vi "创建企业.vi"(9 "企业信息":T2, 11 "数据库操作.i":refnum<class "数据库操作.lvclass">) -> (1 "删除企业成功？":bool, 2 "创建结果":string caption="结果", 3 "数据库操作.o":refnum<class "数据库操作.lvclass">)   [LabVIEW 2013, in "数据库操作.lvclass"]
uses:
  <vilib>/addons/database/Connection.llb/Conn Execute.vi
  <vilib>/Utility/config.llb/Write Key (String).vi
  <vilib>/Utility/config.llb/NI_LVConfig.lvlib
  <vilib>/addons/database/NI_Database_API.lvlib
panel:
  out "剂量统计":enum16{"用户名", "年", "月", "周", "日", "剂量"}(ring)
  out "用户列表":T1(ring)
  out "企业信息.ini":enum16{"登录名", "密码", "企业名称", "邮箱", "电话"}(ring)
  # "字段参考"
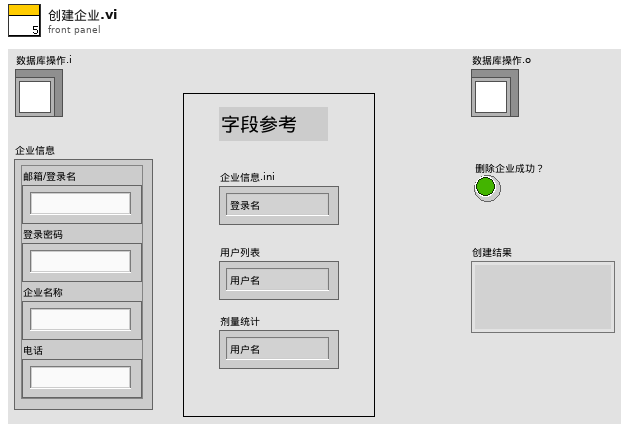
[diagram p1: front panel]
types:
  T1 = enum16{"用户名", "设备MAC", "设备状态", "密码", "职类", "姓名", "电话", "邮箱", "备注", "最后活动"}
  T2 = cluster{"邮箱/登录名":string, "登录密码":string, "企业名称":string, "电话":string}
  T3 = typedef "NI_Database_API.lvlib/Conn ObjectReference.ctl" = refnum<k1>
  T4 = typedef "NI_LVConfig.lvlib/Config Data RefNum.ctl" = refnum<k1>
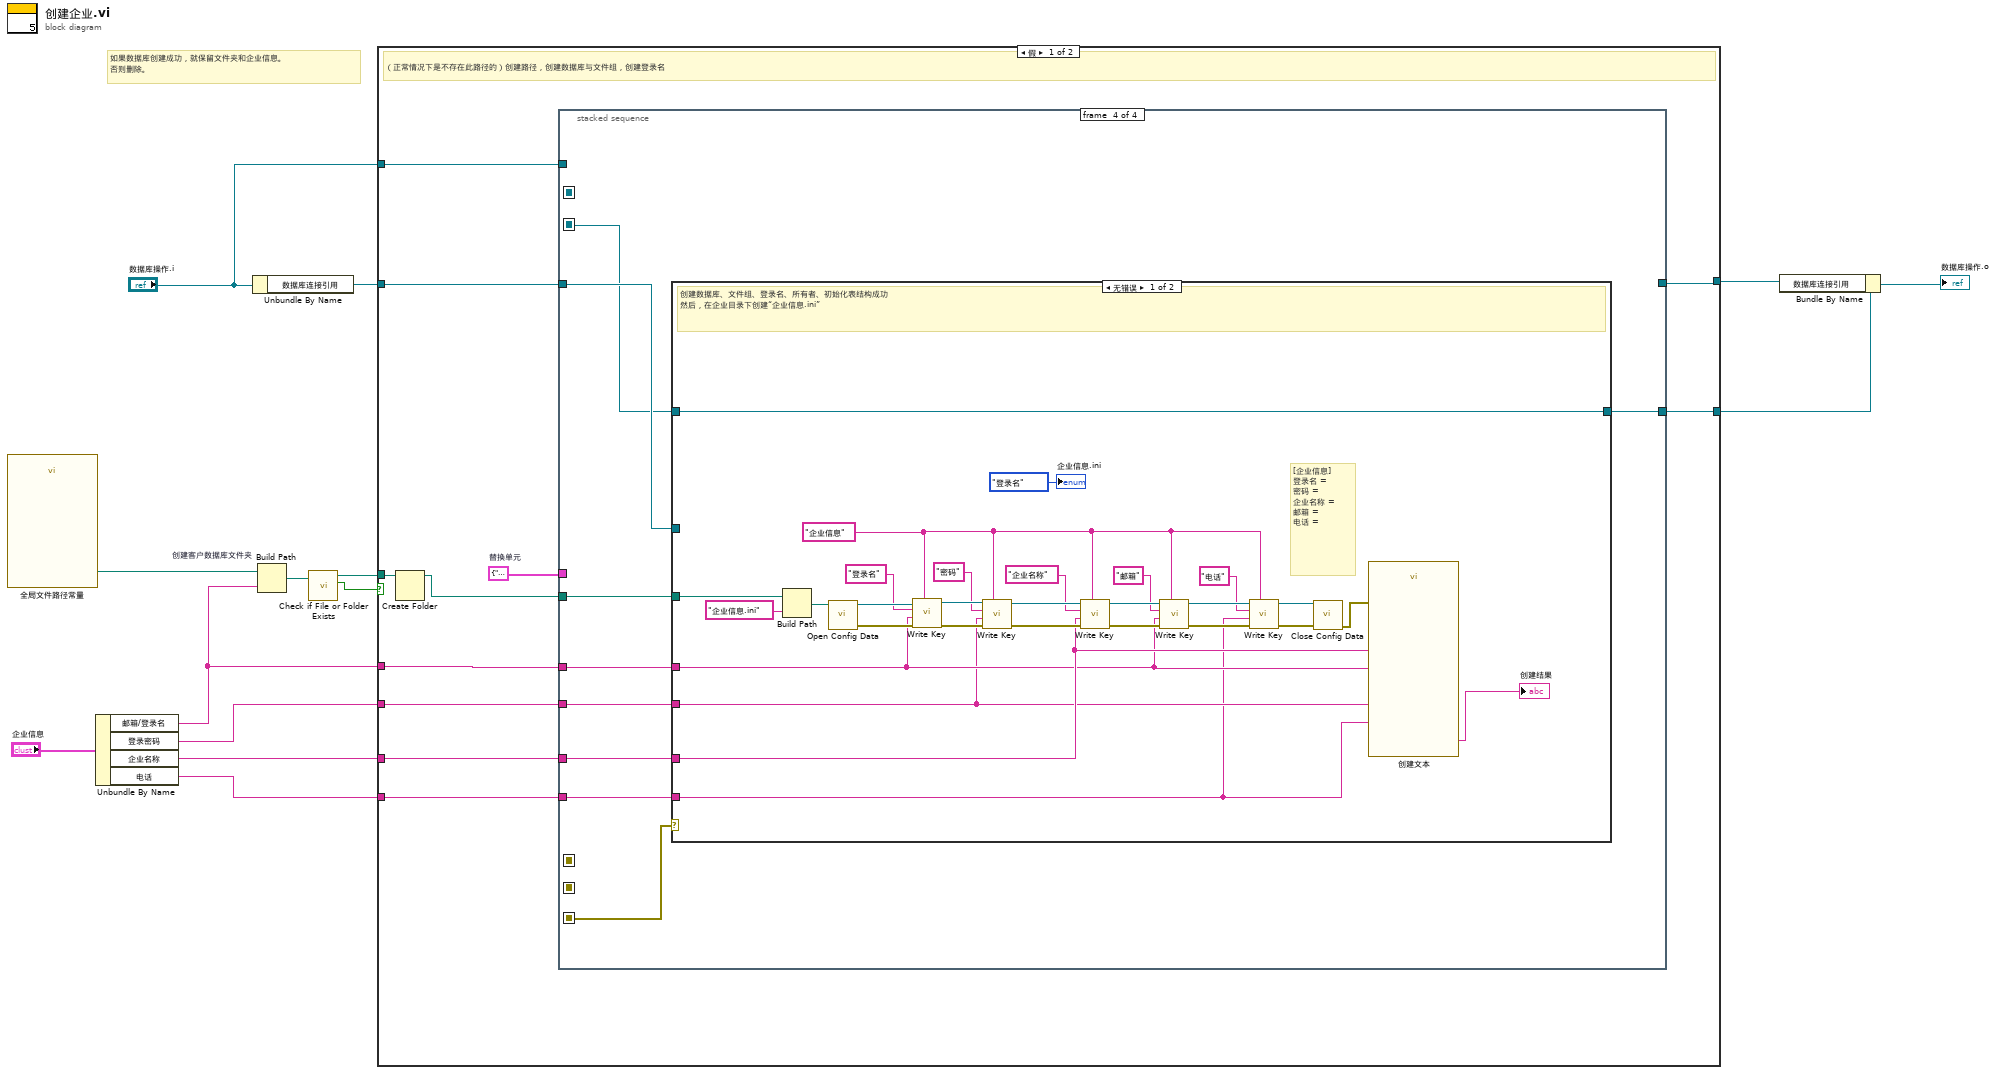
[diagram p0: block diagram]
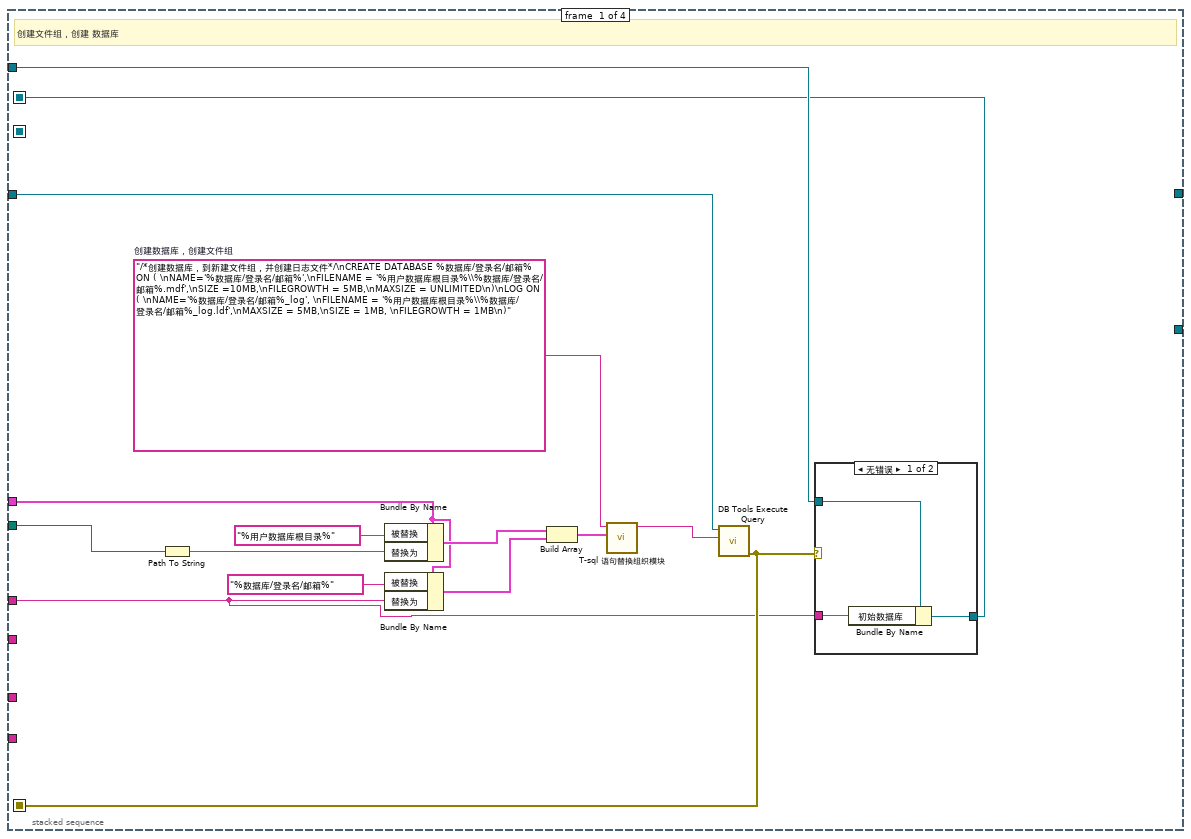
[diagram p2: hidden frame]
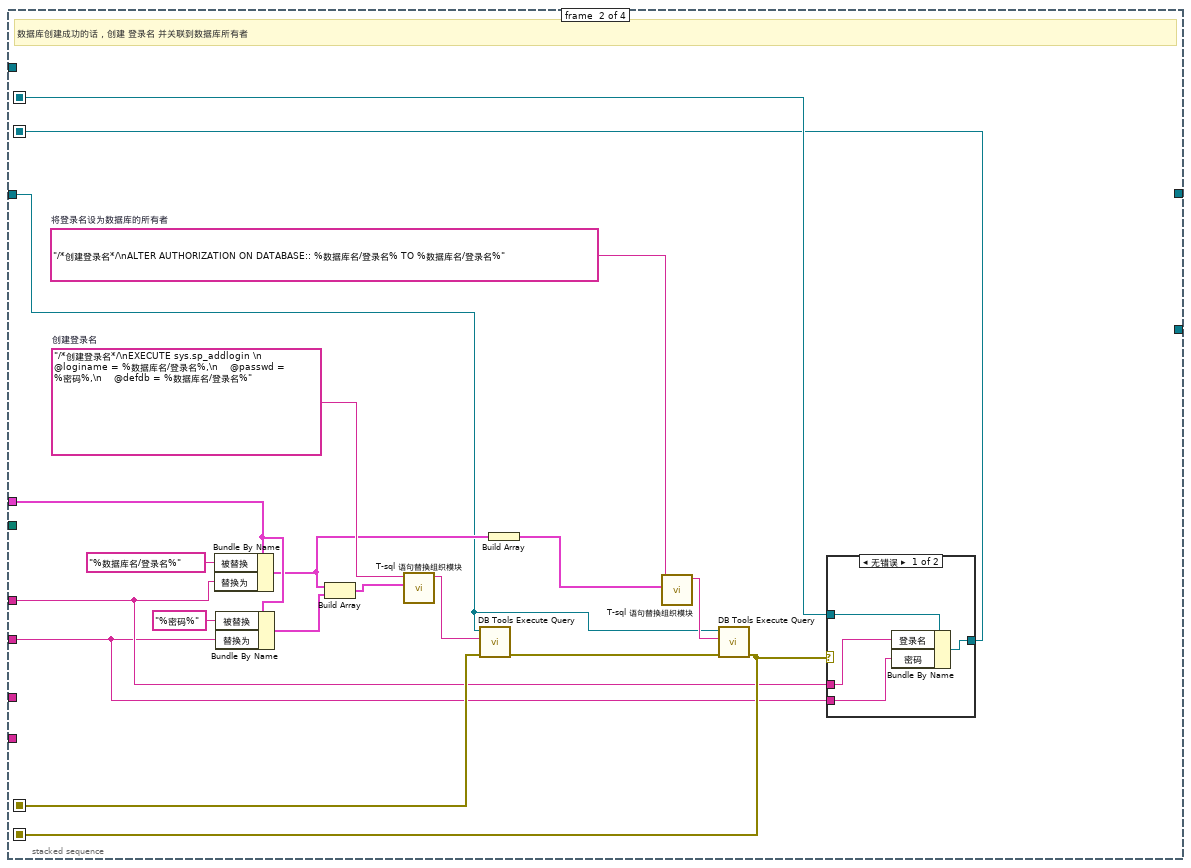
[diagram p4: hidden frame]
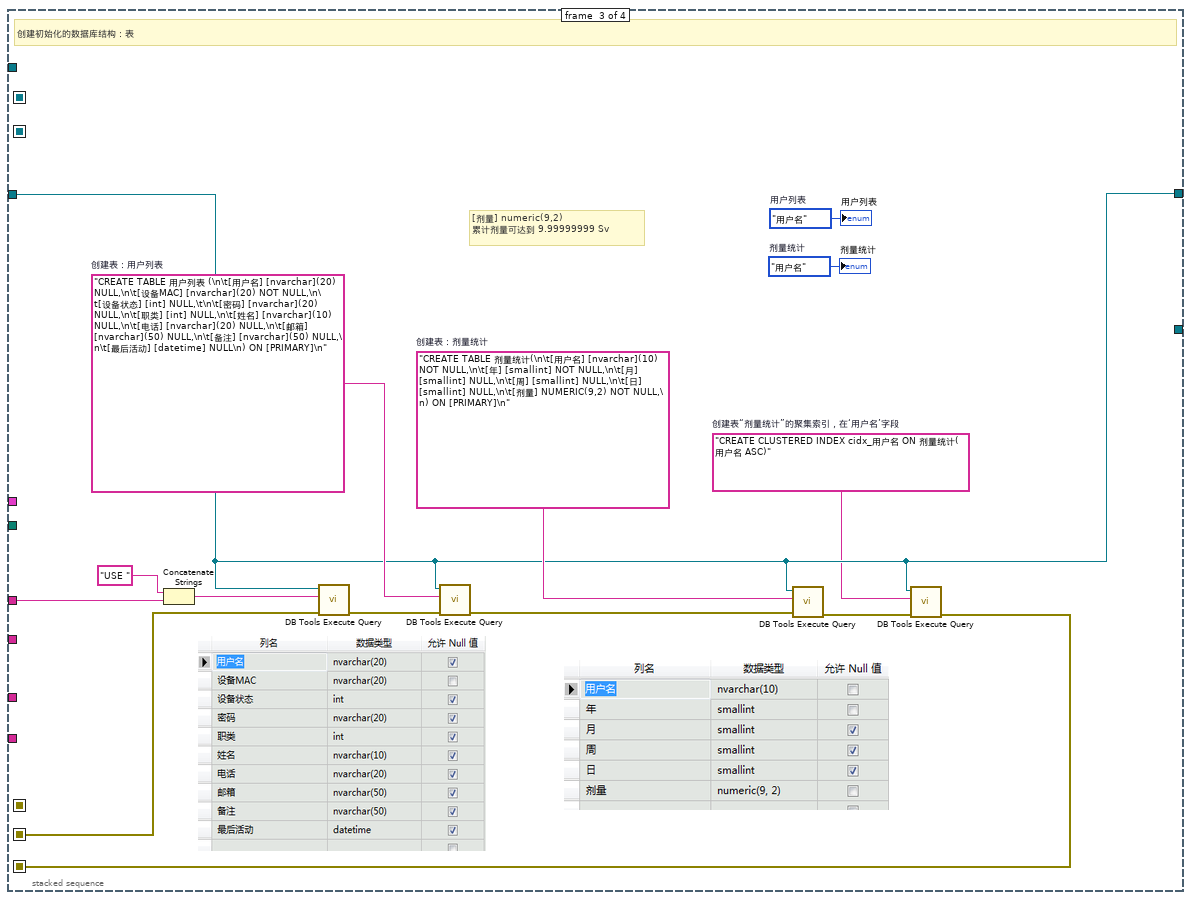
[diagram p6: hidden frame]
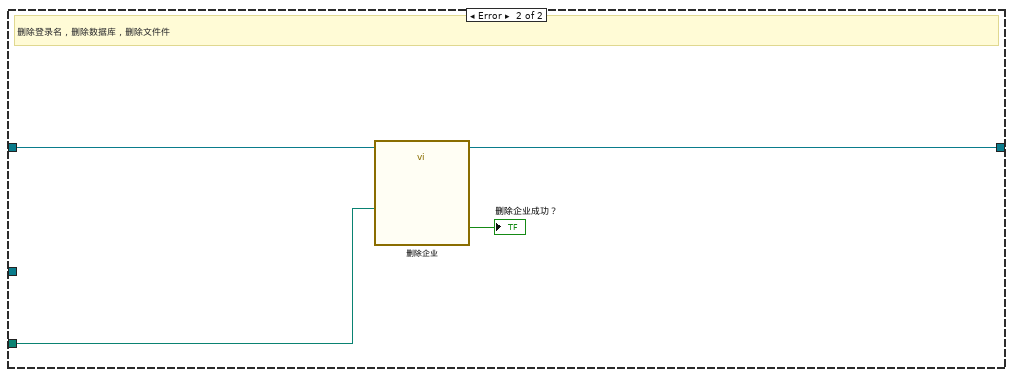
[diagram p7: hidden frame]
diagram:
  # "如果数据库创建成功，就保留文件夹和企业信息。\n否则删除。"
  n1 = call "全局文件路径常量.vi"() -> ("用户数据库根目录"=w14:path)  [unwired: 9 in, 2 out]
  n2 = Unbundle By Name("企业信息") -> ("邮箱/登录名"=w6:string, "登录密码"=w5:string, "企业名称"=w4:string, "电话"=w3:string)
  n3 = Unbundle By Name("数据库操作.i") -> ("数据库连接引用"=w10:T3)
  n4 = Build Path "创建客户数据库文件夹"(base path=w14, name or relative path=w6) -> (appended path=w13:path)
  n5 = call <vilib>:"Check if File or Folder Exists.vi"("path"=w13) -> ("file or folder exists?"=w11:bool, "dup path"=w12:path)  [unwired: 8 in, 1 out]
  n6 = case shown="假" w11 {
    tunnel: w12 -> [w25 _]
    tunnel: w6 -> [w23 _]
    tunnel: w10 -> [w22 w126]
    tunnel: w5 -> [w20 _]
    tunnel: w4 -> [w19 _]
    tunnel: w3 -> [w18 _]
    tunnel: [w17 w126] -> w9
    tunnel: "数据库操作.i" -> [w16 w125]
    tunnel: [w15 w125] -> w1
    frame False {
      w21 = cluster{"被替换":string, "替换为":string} {"被替换"="", "替换为"=""}  # 替换单元
      # "（正常情况下是不存在此路径的）创建路径，创建数据库与文件组，创建登录名"
      n7 = Create Folder(path (use dialog)=w25) -> (created path=w24:path)  [unwired: 2 in, 2 out]
      n8 = stacked-sequence {
        seq-local: [w29 _ _ _] -> [_ w57 _ _]
        seq-local: [_ w49 _ _] -> [_ _ w77 _]
        seq-local: [_ _ w71 _] -> [_ _ _ w91]
        seq-local: [w26 _ _ _] -> [_ w48 _ _]
        seq-local: [_ w45 _ _] -> [_ _ _ w83]
        tunnel: w24 -> [w35 _ _ w89]
        tunnel: w23 -> [w27 w47 w81 w90]
        tunnel: w22 -> [w31 w50 w70 w85]
        tunnel: w21 -> [w30 w55 _ _]
        tunnel: w20 -> [_ w46 _ w88]
        tunnel: w19 -> [_ _ _ w87]
        tunnel: w18 -> [_ _ _ w86]
        tunnel: [_ _ w70 _] -> w17
        tunnel: w16 -> [w28 _ _ _]
        tunnel: [_ _ _ w84] -> w15
        frame #0 {
          w33 = "/*创建数据库，到新建文件组，并创建日志文件*/\nCREATE DATABASE %数据库/登录名/邮箱% ON ( \nNAME='%数据库/登录名/邮箱%',\nFILENAME = '%用户数据库根目录%\\%数据库/登录名/邮箱%.mdf',\nSIZE =10MB,\nFILEGROWTH = 5MB,\nMAXSIZE = UNLIMITED\n)\nLOG ON ( \nNAME='%数据库/登录名/邮箱%_log', \nFILENAME = '%用户数据库根目录%\\%数据库/登录名/邮箱%_log.ldf',\nMAXSIZE = 5MB,\nSIZE = 1MB, \nFILEGROWTH = 1MB\n)"  # 创建数据库，创建文件组
          # "创建文件组，创建 数据库"
          n9 = Path To String(path=w35) -> (string=w38:string)
          n10 = Bundle By Name(cluster=w30, "被替换"="%用户数据库根目录%", "替换为"=w38) -> (w39:cluster{"被替换":string, "替换为":string})
          n11 = Bundle By Name(cluster=w30, "被替换"="%数据库/登录名/邮箱%", "替换为"=w27) -> (w40:cluster{"被替换":string, "替换为":string})
          n12 = Build Array(w39, w40) -> (w34:cluster{"被替换":string, "替换为":string}[])
          n13 = call "T-sql 语句替换组织模块.vi"("替换项"=w34, "T-sql 模板"=w33) -> ("T-sql"=w32:string)  [unwired: 8 in, 1 out]
          n14 = call-poly <vilib>:"DB Tools Execute Query.vi"("SQL query"=w32, "connection reference"=w31) -> ("error out"=w29:errorcluster)  [unwired: 6 in, 1 out]
          n15 = case shown="无错误" w29 {
            tunnel: w28 -> [w43 w44]
            tunnel: w27 -> [w42 _]
            tunnel: [w41 w44] -> w26
            frame No Error {
              n16 = Bundle By Name(cluster=w43, "初始数据库"=w42) -> (w41:refnum<class "数据库操作.lvclass">)
            }
            frame Error {
            }
          }
        }
        frame #1 {
          w54 = "/*创建登录名*/\nALTER AUTHORIZATION ON DATABASE:: %数据库名/登录名% TO %数据库名/登录名%"  # 将登录名设为数据库的所有者
          w59 = "/*创建登录名*/\nEXECUTE sys.sp_addlogin \n    @loginame = %数据库名/登录名%,\n    @passwd = %密码%,\n    @defdb = %数据库名/登录名%"  # 创建登录名
          # "数据库创建成功的话，创建 登录名 并关联到数据库所有者"
          n17 = Bundle By Name(cluster=w55, "被替换"="%数据库名/登录名%", "替换为"=w47) -> (w53:cluster{"被替换":string, "替换为":string})
          n18 = Bundle By Name(cluster=w55, "被替换"="%密码%", "替换为"=w46) -> (w61:cluster{"被替换":string, "替换为":string})
          n19 = Build Array(w53, w61) -> (w60:cluster{"被替换":string, "替换为":string}[])
          n20 = call "T-sql 语句替换组织模块.vi"("替换项"=w60, "T-sql 模板"=w59) -> ("T-sql"=w58:string)  [unwired: 8 in, 1 out]
          n21 = call-poly <vilib>:"DB Tools Execute Query.vi"("error in (no error)"=w57, "SQL query"=w58, "connection reference"=w50) -> ("error out"=w56:errorcluster)  [unwired: 5 in, 1 out]
          n22 = Build Array(w53) -> (w52:cluster{"被替换":string, "替换为":string}[])
          n23 = call "T-sql 语句替换组织模块.vi"("替换项"=w52, "T-sql 模板"=w54) -> ("T-sql"=w51:string)  [unwired: 8 in, 1 out]
          n24 = call-poly <vilib>:"DB Tools Execute Query.vi"("error in (no error)"=w56, "SQL query"=w51, "connection reference"=w50) -> ("error out"=w49:errorcluster)  [unwired: 5 in, 1 out]
          n25 = case shown="无错误" w49 {
            tunnel: w48 -> [w67 w68]
            tunnel: w47 -> [w66 _]
            tunnel: [w65 w68] -> w45
            tunnel: w46 -> [w64 _]
            frame No Error {
              n26 = Bundle By Name(cluster=w67, "登录名"=w66, "密码"=w64) -> (w65:refnum<class "数据库操作.lvclass">)
            }
            frame Error {
            }
          }
        }
        frame #2 {
          w69 = "CREATE CLUSTERED INDEX cidx_用户名 ON 剂量统计( 用户名 ASC)"  # 创建表“剂量统计”的聚集索引，在‘用户名’字段
          w73 = enum16{"用户名", "年", "月", "周", "日", "剂量"}."用户名"  # 剂量统计
          w75 = "CREATE TABLE 剂量统计(\n\t[用户名] [nvarchar](10) NOT NULL,\n\t[年] [smallint] NOT NULL,\n\t[月] [smallint] NULL,\n\t[周] [smallint] NULL,\n\t[日] [smallint] NULL,\n\t[剂量] NUMERIC(9,2) NOT NULL,\n) ON [PRIMARY]\n"  # 创建表：剂量统计
          w74 = T1."用户名"  # 用户列表
          w78 = "CREATE TABLE 用户列表 (\n\t[用户名] [nvarchar](20) NULL,\n\t[设备MAC] [nvarchar](20) NOT NULL,\n\t[设备状态] [int] NULL,\t\n\t[密码] [nvarchar](20) NULL,\n\t[职类] [int] NULL,\n\t[姓名] [nvarchar](10) NULL,\n\t[电话] [nvarchar](20) NULL,\n\t[邮箱] [nvarchar](50) NULL,\n\t[备注] [nvarchar](50) NULL,\n\t[最后活动] [datetime] NULL\n) ON [PRIMARY]\n"  # 创建表：用户列表
          # "[剂量] numeric(9,2)\n累计剂量可达到 9.99999999 Sv"
          # "创建初始化的数据库结构：表"
          n27 = Concatenate Strings("USE " ("SQL query"), w81) -> (w80:string)
          n28 = call-poly <vilib>:"DB Tools Execute Query.vi"("error in (no error)"=w77, "SQL query"=w80, "connection reference"=w70) -> ("error out"=w79:errorcluster)  [unwired: 5 in, 1 out]
          n29 = call-poly <vilib>:"DB Tools Execute Query.vi"("error in (no error)"=w79, "SQL query"=w78, "connection reference"=w70) -> ("error out"=w76:errorcluster)  [unwired: 5 in, 1 out]
          n30 = call-poly <vilib>:"DB Tools Execute Query.vi"("error in (no error)"=w76, "SQL query"=w75, "connection reference"=w70) -> ("error out"=w72:errorcluster)  [unwired: 5 in, 1 out]
          n31 = call-poly <vilib>:"DB Tools Execute Query.vi"("error in (no error)"=w72, "SQL query"=w69, "connection reference"=w70) -> ("error out"=w71:errorcluster)  [unwired: 5 in, 1 out]
          "用户列表" <- w74
          "剂量统计" <- w73
        }
        frame #3 {
          n32 = case shown="无错误" w91 {
            tunnel: w90 -> [w97 _]
            tunnel: w89 -> [w100 w122]
            tunnel: w88 -> [w96 _]
            tunnel: w87 -> [w98 _]
            tunnel: w86 -> [w95 _]
            tunnel: w85 -> [_ _]
            tunnel: w83 -> [w93 w124]
            tunnel: [w93 w123] -> w84
            frame No Error {
              w118 = "企业信息" ("section")
              # "[企业信息]\n登录名 = \n密码 = \n企业名称 = \n邮箱 = \n电话 ="
              # "创建数据库、文件组、登录名、所有者、初始化表结构成功\n然后，在企业目录下创建“企业信息.ini”"
              n33 = Build Path(base path=w100, name or relative path="企业信息.ini" ("名称或相对路径")) -> (appended path=w119:path)
              n34 = call <vilib>:"Open Config Data.vi"("configuration file path"=w119) -> ("error out"=w106:errorcluster, "refnum"=w117:T4)  [unwired: 8 in, 1 out]
              n35 = call-poly <vilib>:"Write Key.vi"("section"=w118, "error in (no error)"=w106, "value"=w97, "key"="登录名" ("section"), "refnum"=w117) -> ("error out"=w105:errorcluster, "refnum out"=w116:T4)  [unwired: 4 in, 1 out]
              n36 = call-poly <vilib>:"Write Key.vi"("section"=w118, "error in (no error)"=w105, "value"=w96, "key"="密码" ("section"), "refnum"=w116) -> ("error out"=w104:errorcluster, "refnum out"=w115:T4)  [unwired: 4 in, 1 out]
              n37 = call-poly <vilib>:"Write Key.vi"("section"=w118, "error in (no error)"=w104, "value"=w98, "key"="企业名称" ("section"), "refnum"=w115) -> ("error out"=w103:errorcluster, "refnum out"=w114:T4)  [unwired: 4 in, 1 out]
              n38 = call-poly <vilib>:"Write Key.vi"("section"=w118, "error in (no error)"=w103, "value"=w97, "key"="邮箱" ("section"), "refnum"=w114) -> ("error out"=w102:errorcluster, "refnum out"=w113:T4)  [unwired: 4 in, 1 out]
              n39 = call-poly <vilib>:"Write Key.vi"("section"=w118, "error in (no error)"=w102, "value"=w95, "key"="电话" ("section"), "refnum"=w113) -> ("error out"=w101:errorcluster, "refnum out"=w112:T4)  [unwired: 4 in, 1 out]
              n40 = call <vilib>:"Close Config Data.vi"("error in (no error)"=w101, "refnum"=w112) -> ("error out"=w94:errorcluster)  [unwired: 8 in, 1 out]
              n41 = call "创建文本"("密码"=w96, "企业名"=w98, "邮箱"=w97, "error in (no error)"=w94, "电话"=w95) -> ("Result"=→"创建结果":string)  [unwired: 9 in, 1 out]
              "企业信息.ini" <- enum16{"登录名", "密码", "企业名称", "邮箱", "电话"}."登录名" ("企业信息")
            }
            frame Error {
              # "删除登录名，删除数据库，删除文件件"
              n42 = call "删除企业.vi"("企业文件夹"=w122, "数据库操作.i"=w124) -> ("删除企业成功？"=→"删除企业成功？":bool, "数据库操作.o"=w123:refnum<class "数据库操作.lvclass">)  [unwired: 8 in]
            }
          }
        }
      }
    }
    frame True {
    }
  }
  n43 = Bundle By Name(cluster=w1, "数据库连接引用"=w9) -> (→"数据库操作.o":refnum<class "数据库操作.lvclass">)
